vi "查找二维数组.vi"(1 "数值":i32, 2 "数组":i32[][](array[numeric])) -> (0 "索引":i32)   [LabVIEW 2017]
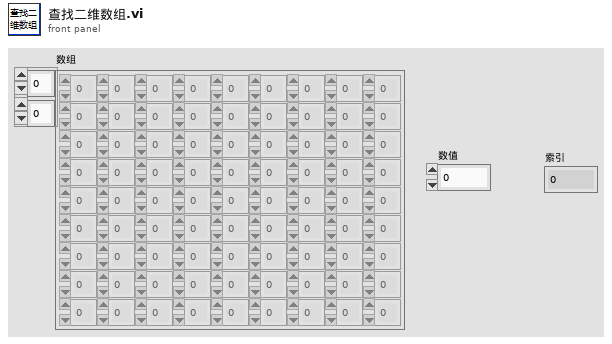
[diagram p1: front panel]
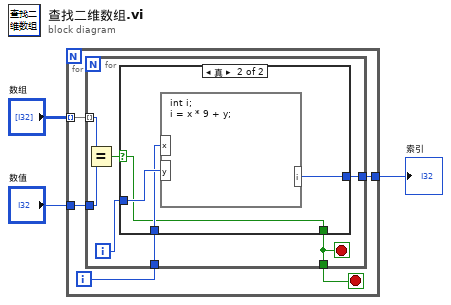
[diagram p0: block diagram]
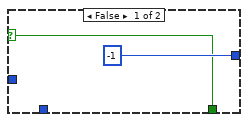
[diagram p2: hidden frame]
diagram:
  n1 = for {
    tunnel: "数组" -> [w8] mode=indexing
    tunnel: "数值" -> [w7]
    tunnel: [w6] -> w1
    i -> [w5]
    stop <- w4 stop-if-true
    n2 = for {
      tunnel: w8 -> [w15] mode=indexing
      tunnel: w7 -> [w14]
      tunnel: [w12] -> w6
      tunnel: w5 -> [w10]
      tunnel: [w9] -> w4
      i -> [w11]
      stop <- w9 stop-if-true
      n3 = Equal?(x=w15, y=w14) -> (x = y?=w13:bool)
      n4 = case shown="真" w13 {
        selector: w13 -> [w16 w18]
        tunnel: [-1 w21] -> w12
        tunnel: w11 -> [_ w20]
        tunnel: w10 -> [_ w19]
        tunnel: [w16 w18] -> w9
        frame False {
        }
        frame True {
          n5 = formula code="int i;\ni = x * 9 + y;"("x"=w19, "y"=w20) -> ("i"=w21:i32)
        }
      }
    }
  }
  "索引" <- w1
